vi "Cycle Begin.vi"(8 "error in (no error)":errorcluster, 11 "Framework in":refnum<class "Framework.lvclass">) -> (0 "error out":errorcluster, 3 "Framework out":refnum<class "Framework.lvclass">)   [LabVIEW 2019, in "DSF Core.lvlib" / "Framework.lvclass"]
uses:
  Framework.lvclass
  Framework.lvclass/Framework.ctl
  Performance/Performance.lvclass/Performance.ctl
  Plugin/Plugin.lvclass/Plugin.ctl
  Timing/Timing.lvclass/Timing.ctl
  Transfer Group/Transfer Group.lvclass/Transfer Group.ctl
  Plugin/Is Active.vi
  Plugin/Set Active.vi
  Plugin/Active Transfer Groups.vi
  Timing/Is Active Cycle.vi
  Transfer Group/Is Active.vi
  Transfer Group/Set Active.vi
  Plugin/Iteration.vi
  Timing/Get Decimation.vi
  Timing/Get Offset.vi
  Plugin/Get Timing.vi
  Timing/Get Iteration.vi
  Performance/Performance.lvclass
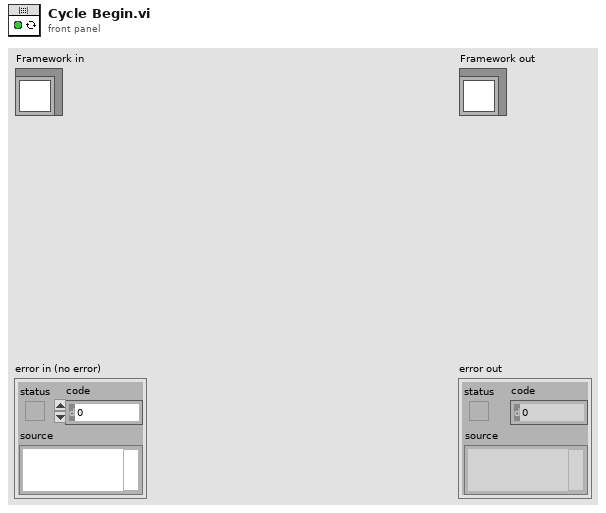
[diagram p1: front panel]
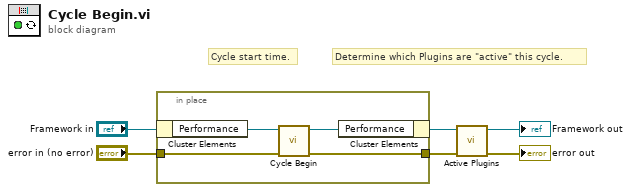
[diagram p0: block diagram]
diagram:
  # "Determine which Plugins are \"active\" this cycle."
  # "Cycle start time."
  n1 = in-place {
    in-place-border: "error in (no error)" -> [w8]
    in-place-border: [w7] -> w3
    n2 = in-place-cluster #1("Framework in") -> ("Performance"=w10:refnum<class "Performance.lvclass">)
    n3 = call "Cycle Begin.vi"("error in (no error)"=w8, "Performance in"=w10) -> ("error out"=w7:errorcluster, "Performance out"=w9:refnum<class "Performance.lvclass">)  [unwired: 8 in]
    n4 = in-place-cluster #1("Performance"=w9) -> (w4:refnum<class "Framework.lvclass">)
  }
  n5 = call "Active Plugins.vi"("error in (no error)"=w3, "Framework in"=w4) -> ("error out"=→"error out":errorcluster, "Framework out"=→"Framework out":refnum<class "Framework.lvclass">)  [unwired: 8 in]
